vi "getChannelValues.vi"(8 "error in (no error)":errorcluster, 10 "channel_type":enum16{"ao", "do", "ai", "di", "rf"}(ring), 11 "StaticOutputEditor in":refnum<class "StaticOutputEditor.lvclass">) -> (0 "error out":errorcluster, 3 "StaticOutputEditor out":refnum<class "StaticOutputEditor.lvclass">)   [LabVIEW 2009, in "Views.lvlib" / "ScriptEditor.lvlib" / "StaticOutputEditor.lvclass"]
uses:
  StaticOutputEditor.lvclass
  StaticOutputEditor.lvclass/StaticOutputEditor.ctl
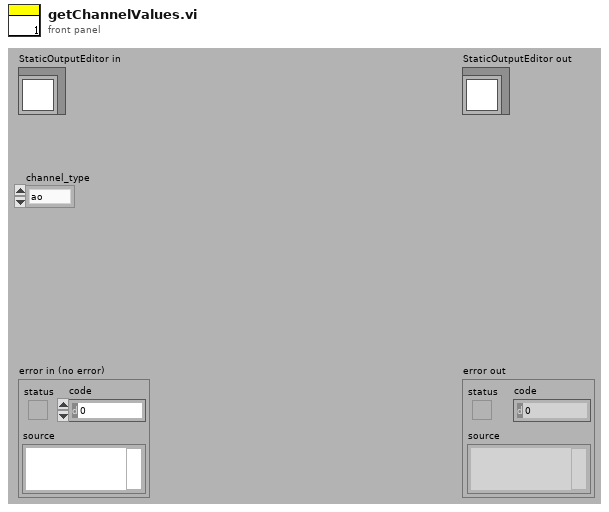
[diagram p1: front panel]
types:
  T1 = cluster{"channelName":string, "value":string, "freq":string, "phase":string}[]
  T2 = cluster{"channelName":string, "value":string, "freq":string, "phase":string}
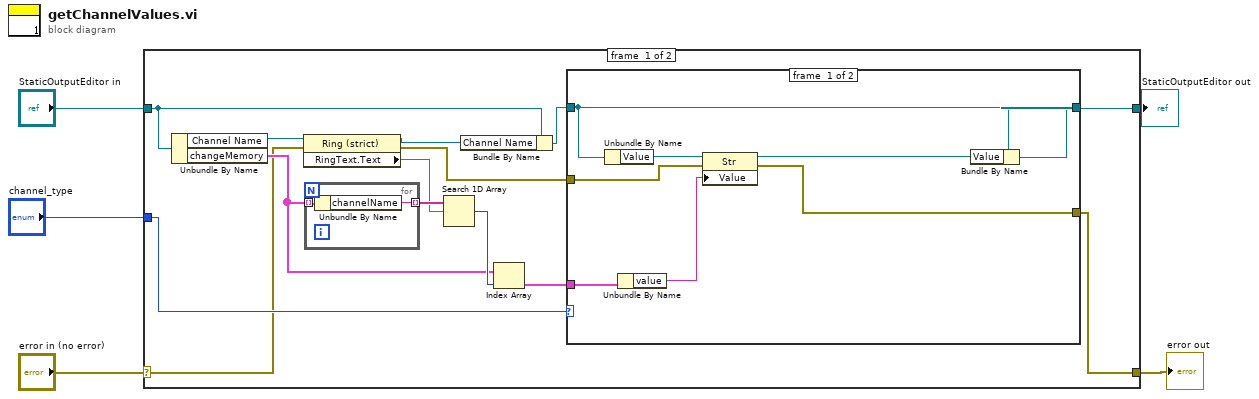
[diagram p0: block diagram]
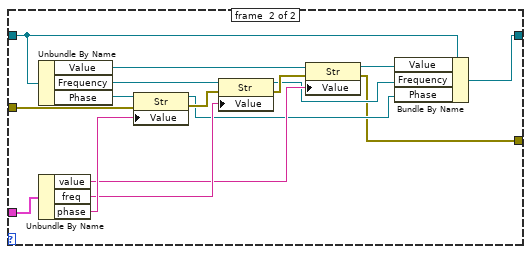
[diagram p2: hidden frame]
diagram:
  n1 = case shown="No Error" "error in (no error)" {
    selector: "error in (no error)" -> [w7 w47]
    tunnel: [w6 w47] -> w4
    tunnel: [w13 w46] -> w2
    tunnel: "StaticOutputEditor in" -> [w11 w46]
    tunnel: "channel_type" -> [w14 _]
    frame #0 {
      n2 = Unbundle By Name(w11) -> ("Channel Name"=w19:refnum<vi>, "changeMemory"=w15:T1)
      n3 = property class="Ring (strict)"(reference=w19, error in=w7) -> (reference out=w12:refnum<vi>, error out=w8:errorcluster, "RingText.Text"=w17:string)
      n4 = for {
        tunnel: w15 -> [w45] mode=indexing
        tunnel: [w44] -> w18 mode=indexing
        n5 = Unbundle By Name(w45) -> ("channelName"=w44:string)
      }
      n6 = Search 1D Array(1D array=w18, element=w17) -> (index of element=w16:i32)  [unwired: 1 in]
      n7 = Bundle By Name(cluster=w11, "Channel Name"=w12) -> (w10:refnum<class "StaticOutputEditor.lvclass">)
      n8 = Index Array(array=w15, index=w16) -> (element=w9:T2)
      n9 = case shown="\"ao\", Default" w14 {
        tunnel: w10 -> [w23 w34]
        tunnel: [w22 w28] -> w13
        tunnel: w9 -> [w27 w40]
        tunnel: [w20 w30] -> w6
        tunnel: w8 -> [w26 w29]
        frame #0 {
          n10 = Unbundle By Name(w23) -> ("Value"=w25:refnum<vi>)
          n11 = Unbundle By Name(w27) -> ("value"=w24:string)
          n12 = property class="Str"(reference=w25, error in=w26, "Value"=w24) -> (reference out=w21:refnum<vi>, error out=w20:errorcluster)
          n13 = Bundle By Name(cluster=w23, "Value"=w21) -> (w22:refnum<class "StaticOutputEditor.lvclass">)
        }
        frame #1 {
          n14 = Unbundle By Name(w34) -> ("Value"=w43:refnum<vi>, "Frequency"=w42:refnum<vi>, "Phase"=w41:refnum<vi>)
          n15 = Unbundle By Name(w40) -> ("value"=w37:string, "freq"=w38:string, "phase"=w39:string)
          n16 = property class="Str"(reference=w41, error in=w29, "Value"=w39) -> (reference out=w31:refnum<vi>, error out=w35:errorcluster)
          n17 = property class="Str"(reference=w42, error in=w35, "Value"=w38) -> (reference out=w32:refnum<vi>, error out=w36:errorcluster)
          n18 = property class="Str"(reference=w43, error in=w36, "Value"=w37) -> (reference out=w33:refnum<vi>, error out=w30:errorcluster)
          n19 = Bundle By Name(cluster=w34, "Value"=w33, "Frequency"=w32, "Phase"=w31) -> (w28:refnum<class "StaticOutputEditor.lvclass">)
        }
      }
    }
    frame #1 {
    }
  }
  "error out" <- w4
  "StaticOutputEditor out" <- w2
